vi "qrread-2.vi"() -> ()   [LabVIEW 2019]
uses:
  <vilib>/vision/Instrument.llb/QR Code Report.ctl
  <vilib>/vision/Instrument.llb/QR Code Model Type.ctl
  <vilib>/vision/Instrument.llb/QR Code Stream Mode Type.ctl
  <vilib>/vision/Instrument.llb/Data Matrix Polarity.ctl
  <vilib>/vision/Instrument.llb/Demodulation Mode.ctl
  <vilib>/vision/Instrument.llb/Cell Sample Size.ctl
  <vilib>/vision/Instrument.llb/Cell Filter Mode.ctl
  Global 1.vi
panel:
  in  "Stop (F) in":bool caption="Stop (F)"
  out "t":i32
  out "Array":bool[](array[boolean])
  out "appended array":bool[](array[boolean])
  out "Found?":bool
  out "Bounding Box":cluster{"x":sgl, "y":sgl}[](array[cluster])
  out "QR Barcode Report (2D Barcode Reader 1)":T1={"Found?"=FALSE, "Data"="", "Bounding Box"=[], "Errors Corrected"=0, "Dimensions (Rows/Cols)"=0, "Version"=0, "QR Model"=3, "Stream Mode"=0, "Barcode Polarity"=-2, "Mirrored?"=FALSE, "Append Stream Position"=0, "Size of Append Stream"=0, "First EAN-128 ID"=0, "First Alternate Language ID"=0, "Append Stream ID"=0, "Minimum Edge Strength"=30, "Demodulation Mode"=-2, "Cell Sample Size"=-2, "Cell Filter Mode"=-2} {"Append Stream ID" format="%x"; "Cell Filter Mode" items=["Auto-detect"=-2, "Average"=0, "Median"=1, "Central Average"=2, "High Average"=3, "Low Average"=4, "Very High Average"=5, "Very Low Average"=6, "All Filters"=8]; "Cell Sample Size" items=["Auto-detect"=-2, "1x1"=1, "2x2"=2, "3x3"=3, "4x4"=4, "5x5"=5, "6x6"=6, "7x7"=7]; "Demodulation Mode" items=["Auto-detect"=-2, "Histogram"=0, "Local Contrast"=1, "Combination"=2, "All"=3]; "Barcode Polarity" items=["Auto-detect"=-2, "Black on White"=0, "White on Black"=1]; "Stream Mode" items=["Auto-detect", "Numeric", "AlphaNumeric", "Mixed", "Raw Bytes", "UCC/EAN-128 - In Tokens", "UCC/EAN-128 - In Data", "Extended Character Interpretation", "Kanji"]; "QR Model" items=["Auto Detect", "Micro", "Model 1", "Model 2"]; "Version" max=40 step=1}
  in  "Stop (F)":bool
  out "Image Out":T8(plugin-control)
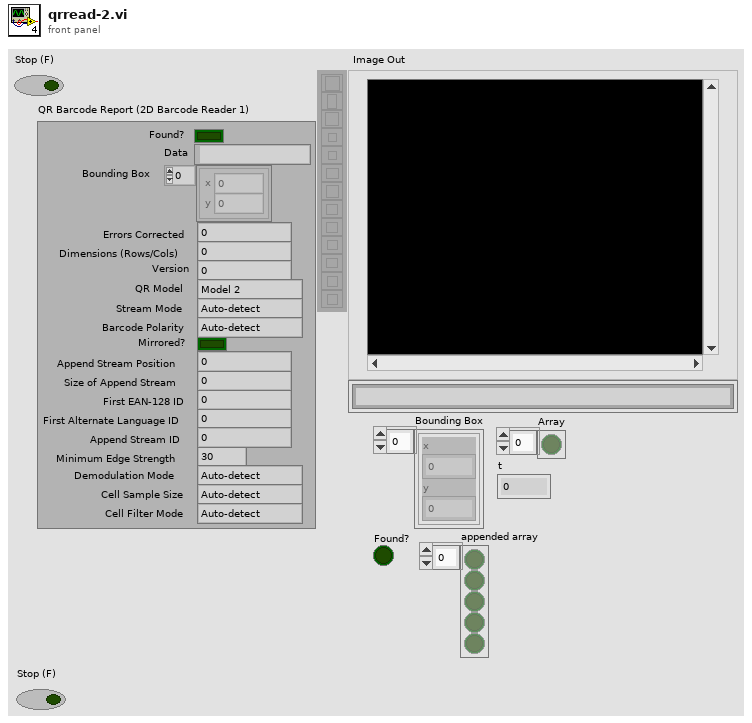
[diagram p1: front panel]
types:
  T1 = typedef "QR Code Report.ctl" = cluster{"Found?":bool, "Data":string, "Bounding Box":cluster{"x":sgl, "y":sgl}[], "Errors Corrected":u32, "Dimensions (Rows/Cols)":u32, "Version":u32, "QR Model":T2, "Stream Mode":T3, "Barcode Polarity":T4, "Mirrored?":bool, "Append Stream Position":u32, "Size of Append Stream":u32, "First EAN-128 ID":i32, "First Alternate Language ID":i32, "Append Stream ID":u32, "Minimum Edge Strength":u32, "Demodulation Mode":T5, "Cell Sample Size":T6, "Cell Filter Mode":T7}
  T2 = typedef "QR Code Model Type.ctl" = i32
  T3 = typedef "QR Code Stream Mode Type.ctl" = i32
  T4 = typedef "Data Matrix Polarity.ctl" = i32
  T5 = typedef "Demodulation Mode.ctl" = i32
  T6 = typedef "Cell Sample Size.ctl" = i32
  T7 = typedef "Cell Filter Mode.ctl" = i32
  T8 = typedef "IMAQ Image.ctl" = refnum<image>
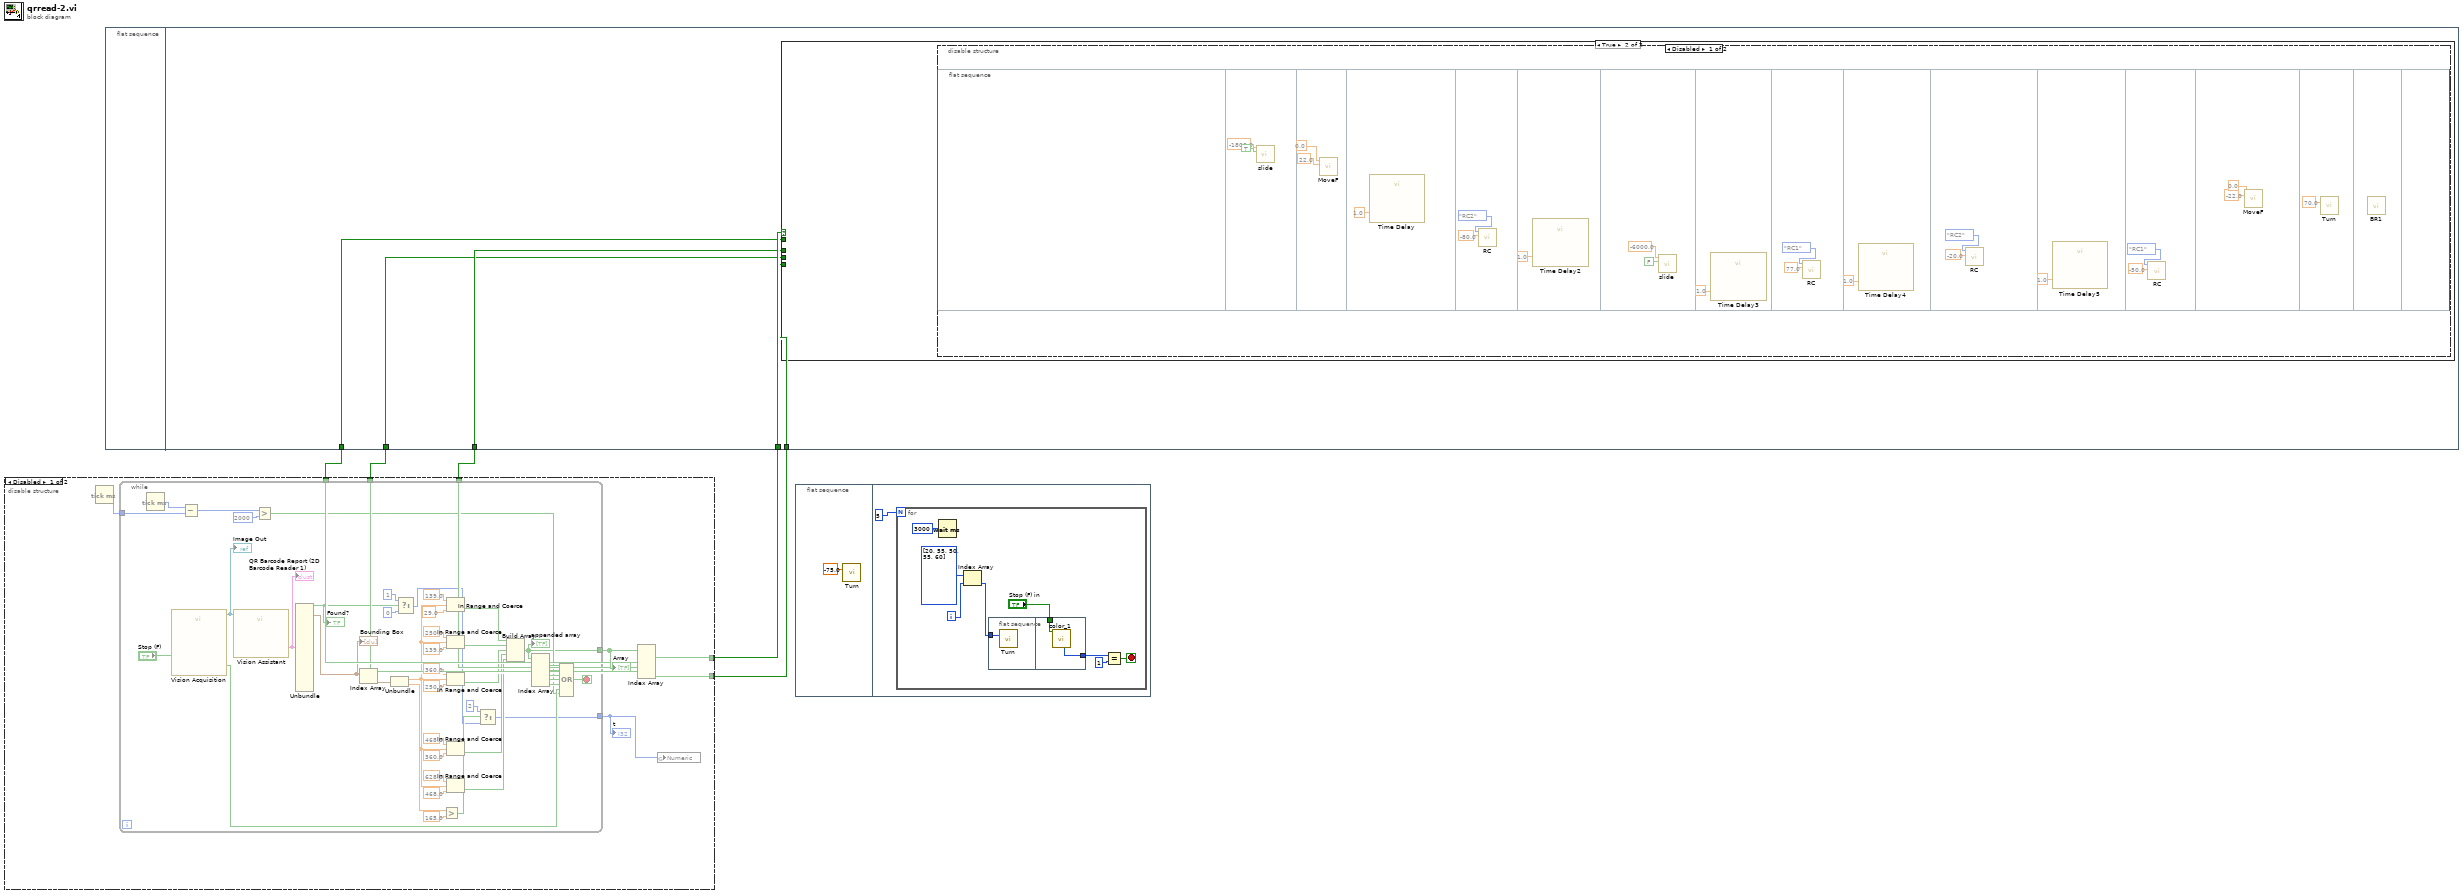
[diagram p0: block diagram]
diagram:
  n1 = disable-structure shown="Disabled" {
    disable-tunnel: [w10 _] -> w5
    disable-tunnel: [w9 _] -> w4
    disable-tunnel: [w8 _] -> w3
    disable-tunnel: [w7 _] -> w2
    disable-tunnel: [w6 _] -> w1
    frame Disabled {
      n2 = Tick Count (ms)() -> (millisecond timer value=w11:u32)
      n3 = while {
        tunnel: w11 -> [w36]
        tunnel: [w25] -> w12
        tunnel: [w16] -> w13
        stop <- w26 stop-if-true
        n4 = Tick Count (ms)() -> (millisecond timer value=w37:u32)
        n5 = call "Vision Acquisition"("Stop (F)"="Stop (F)") -> ("Image Out"=w15:T8, "Stopped"=w28:bool)  [unwired: 24 in, 1 out]
        "Image Out" <- w15
        n6 = Subtract(x=w37, y=w36) -> (x-y=w35:u32)
        n7 = call "Vision Assistant"("Image In"=w15) -> ("QR Barcode Report (2D Barcode Reader 1)"=w14:T1)  [unwired: 24 in, 2 out]
        "QR Barcode Report (2D Barcode Reader 1)" <- w14
        n8 = Greater?(x=w35, y=u32 2000) -> (0:w27:bool)
        n9 = Unbundle(w14) -> ("Found?"=w21:bool, "Bounding Box"=w55:cluster{"x":sgl, "y":sgl}[])  [unwired: 17 out]
        "Bounding Box" <- w55
        "Found?" <- w21
        n10 = Index Array(array=w55) -> (element=w44:cluster{"x":sgl, "y":sgl})  [unwired: 1 in]
        n11 = Unbundle(w44) -> ("x"=w43:sgl, "y"=w24:sgl)
        n12 = Select(t=1, s=w21, f=0) -> (s? t:f=w18:i32)
        n13 = Greater?(x=w24, y=sgl 165.0) -> (0:w22:bool)
        n14 = In Range and Coerce(upper limit=139.0, x=w43, lower limit=29.0) -> (In Range?=w42:bool)  [unwired: 1 out]
        n15 = In Range and Coerce(upper limit=250.0, x=w43, lower limit=139.0) -> (In Range?=w41:bool)  [unwired: 1 out]
        n16 = In Range and Coerce(upper limit=360.0, x=w43, lower limit=250.0) -> (In Range?=w40:bool)  [unwired: 1 out]
        n17 = In Range and Coerce(upper limit=468.0, x=w43, lower limit=360.0) -> (In Range?=w39:bool)  [unwired: 1 out]
        n18 = In Range and Coerce(upper limit=628.0, x=w43, lower limit=468.0) -> (In Range?=w38:bool)  [unwired: 1 out]
        n19 = Select(t=2, s=w22, f=w18) -> (s? t:f=w16:i32)
        n20 = Build Array(w42, w41, w40, w39, w38) -> (w25:bool[])
        "appended array" <- w25
        n21 = Index Array(array=w25) -> (element #1=w33:bool, element #2=w32:bool, element #3=w31:bool, element #4=w30:bool, element #5=w29:bool)  [unwired: 5 in]
        n22 = Compound Arithmetic op=OR(w33, w32, w31, w30, w29, w28, w27) -> (w26:bool)
      }
      "Array" <- w12
      "t" <- w13
      n23 = Index Array(array=w12) -> (element #1=w10:bool, element #2=w9:bool, element #3=w8:bool, element #4=w7:bool, element #5=w6:bool)  [unwired: 5 in]
      n24 = global write "Global 1.vi" "Numeric"(w13) -> ()
    }
    frame Enabled {
    }
  }
  n25 = flat-sequence {
    tunnel: w5 -> [w61]
    tunnel: w4 -> [w60]
    tunnel: w3 -> [w59]
    tunnel: w2 -> [w58]
    tunnel: w1 -> [w57]
    frame #0 {
    }
    frame #1 {
      n26 = case shown="True" w61 {
        tunnel: w60 -> [w65 _]
        tunnel: w59 -> [w64 _]
        tunnel: w58 -> [w63 _]
        tunnel: w57 -> [w62 _]
        frame False {
          n27 = case shown="False" w65 {
            tunnel: w64 -> [w68 _]
            tunnel: w63 -> [w67 _]
            tunnel: w62 -> [w66 _]
            frame False {
              n28 = case shown="False" w68 {
                tunnel: w67 -> [w70 _]
                tunnel: w66 -> [w69 _]
                frame False {
                  n29 = case shown="False" w70 {
                    tunnel: w69 -> [w71 _]
                    frame False {
                      n30 = case shown="True" w71 {
                        frame False {
                        }
                        frame True {
                        }
                      }
                    }
                    frame True {
                    }
                  }
                }
                frame True {
                }
              }
            }
            frame True {
            }
          }
        }
        frame True {
          n31 = disable-structure shown="Disabled" {
            frame Disabled {
              n32 = flat-sequence {
                frame #0 {
                }
                frame #1 {
                  n33 = call "slide.vi"("Reset Counter"=TRUE, "Numeric"=-1800.0) -> ()  [unwired: 7 in, 3 out]
                }
                frame #2 {
                  n34 = call "MoveF.vi"("X"=0.0, "Y"=22.0) -> ()  [unwired: 13 in, 1 out]
                }
                frame #3 {
                  n35 = call "Time Delay"("Delay Time (s)"=1.0) -> ()  [unwired: 10 in, 1 out]
                }
                frame #4 {
                  n36 = call "RC.vi"("數值"=-80.0, "選擇RC"=enum16{"請選擇RC", "RC1", "RC2", "RC3"}."RC2") -> ()  [unwired: 9 in, 1 out]
                }
                frame #5 {
                  n37 = call "Time Delay2"("Delay Time (s)"=1.0) -> ()  [unwired: 10 in, 1 out]
                }
                frame #6 {
                  n38 = call "slide.vi"("Reset Counter"=FALSE, "Numeric"=-6000.0) -> ()  [unwired: 7 in, 3 out]
                }
                frame #7 {
                  n39 = call "Time Delay3"("Delay Time (s)"=1.0) -> ()  [unwired: 10 in, 1 out]
                }
                frame #8 {
                  n40 = call "RC.vi"("數值"=77.0, "選擇RC"=enum16{"請選擇RC", "RC1", "RC2", "RC3"}."RC1") -> ()  [unwired: 9 in, 1 out]
                }
                frame #9 {
                  n41 = call "Time Delay4"("Delay Time (s)"=1.0) -> ()  [unwired: 10 in, 1 out]
                }
                frame #10 {
                  n42 = call "RC.vi"("數值"=-20.0, "選擇RC"=enum16{"請選擇RC", "RC1", "RC2", "RC3"}."RC2") -> ()  [unwired: 9 in, 1 out]
                }
                frame #11 {
                  n43 = call "Time Delay5"("Delay Time (s)"=1.0) -> ()  [unwired: 10 in, 1 out]
                }
                frame #12 {
                  n44 = call "RC.vi"("數值"=-50.0, "選擇RC"=enum16{"請選擇RC", "RC1", "RC2", "RC3"}."RC1") -> ()  [unwired: 9 in, 1 out]
                }
                frame #13 {
                  n45 = call "MoveF.vi"("X"=0.0, "Y"=-22.0) -> ()  [unwired: 13 in, 1 out]
                }
                frame #14 {
                  n46 = call "Turn.vi"("角度"=70.0) -> ()  [unwired: 14 in, 1 out]
                }
                frame #15 {
                  n47 = call "BR1.vi"() -> ()  [unwired: 11 in, 1 out]
                }
                frame #16 {
                }
              }
            }
            frame Enabled {
            }
          }
        }
      }
    }
  }
  n48 = flat-sequence {
    frame #0 {
      n49 = call "Turn.vi"("角度"=-75.0) -> ()  [unwired: 14 in, 1 out]
    }
    frame #1 {
      n50 = for {
        N: 5 -> [_]
        i -> [w97]
        stop <- w99 stop-if-true
        n51 = Wait (ms)(milliseconds to wait=u32 3000) -> ()  [unwired: 1 out]
        n52 = Index Array(array=i32[] [20, 55, 50, 55, 60], index=w97) -> (element=w102:i32)
        n53 = flat-sequence {
          tunnel: w102 -> [w104]
          tunnel: [w106] -> w98
          tunnel: "Stop (F) in" -> [w105]
          frame #0 {
            n54 = call "Turn.vi"("角度"=w104) -> ()  [unwired: 14 in, 1 out]
          }
          frame #1 {
            n55 = call "color_1.vi"("Stop (F) in"=w105) -> ("yellow"=w106:i32)  [unwired: 3 in, 7 out]
          }
        }
        n56 = Equal?(x=w98, y=1) -> (x = y?=w99:bool)
      }
    }
  }
